vi "Get Common Doc Dir.vi"(11 "Project XML Editor in":refnum<class "Project XML Editor.lvclass">) -> (2 "Common Doc Dir":string, 3 "Project XML Editor out":refnum<class "Project XML Editor.lvclass">)   [LabVIEW 2020, in "LVLIBP CD XML Updater.lvlib" / "Project XML Editor.lvclass"]
uses:
  Project XML Editor.lvclass
  Project XML Editor.lvclass/Project XML Editor.ctl
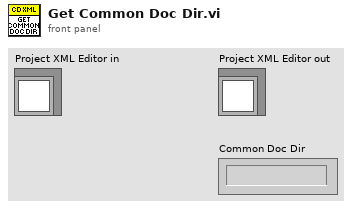
[diagram p1: front panel]
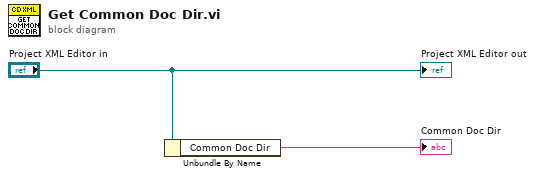
[diagram p0: block diagram]
diagram:
  n1 = Unbundle By Name("Project XML Editor in") -> ("Common Doc Dir"=→"Common Doc Dir":string)
  "Project XML Editor out" <- "Project XML Editor in"
